vi "Handle Command.vi"(8 "error in (no error)":errorcluster, 9 "Data":variant, 10 "Command":string, 11 "Inst.TSL210 in":refnum<class "Inst.TSL210.lvclass">) -> (0 "error out":errorcluster, 1 "Processed Data":variant, 2 "Command":string, 3 "Inst.TSL210 out":refnum<class "Inst.TSL210.lvclass">)   [LabVIEW 2019, in "Inst.TSL210.lvclass"]
uses:
  Inst.TSL210.lvclass
  Inst.TSL210.lvclass/Inst.TSL210.ctl
  <userlib>/LevyLab/Instrument Framework/Instrument Types/VSource/Instrument.VSource.lvclass
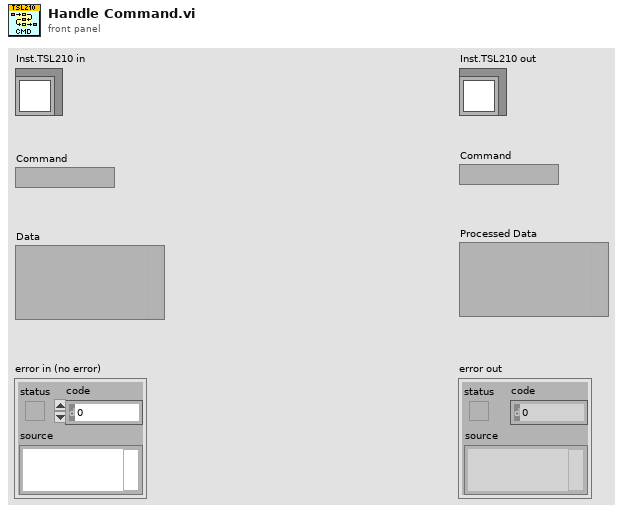
[diagram p1: front panel]
types:
  T1 = typedef "Inst.TSL210.lvclass/Inst.TSL210.getAll--Cluster.ctl" = cluster{"Wavelength (nm)":dbl, "Power (mW)":dbl, "Status: LD":bool, "Status: COH":bool, "Status: TempError":bool, "Status: CurrentLimit":bool, "Status: SystemBusy":bool, "Status: ATT":bool, "Status: ACC":bool, "Status: FT":bool}
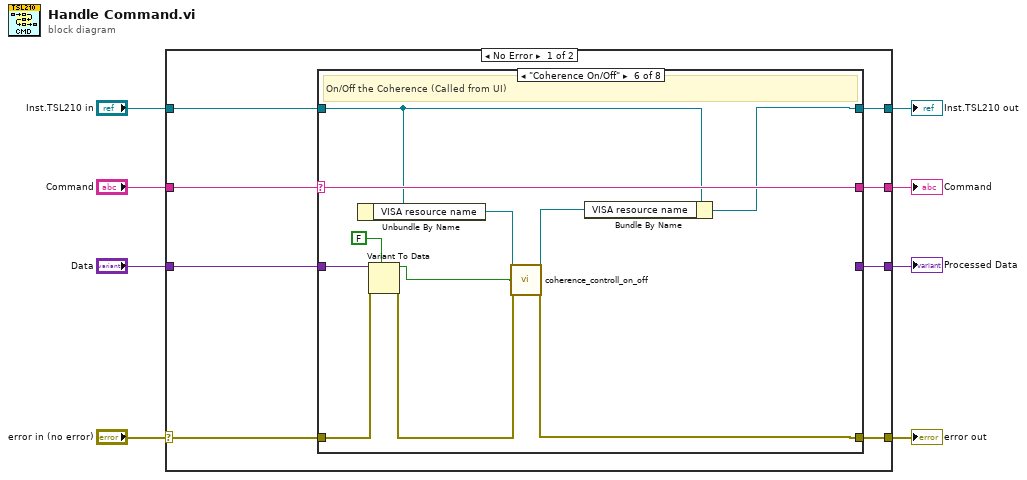
[diagram p0: block diagram]
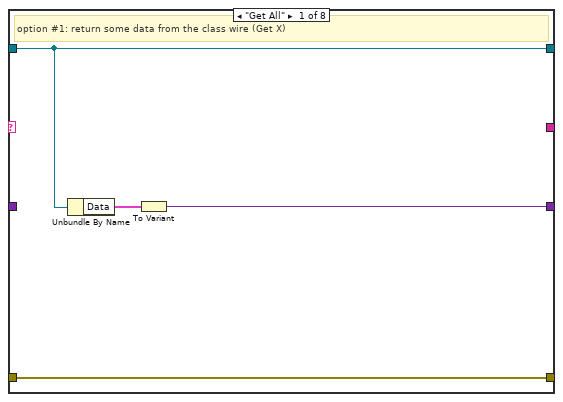
[diagram p2: hidden frame]
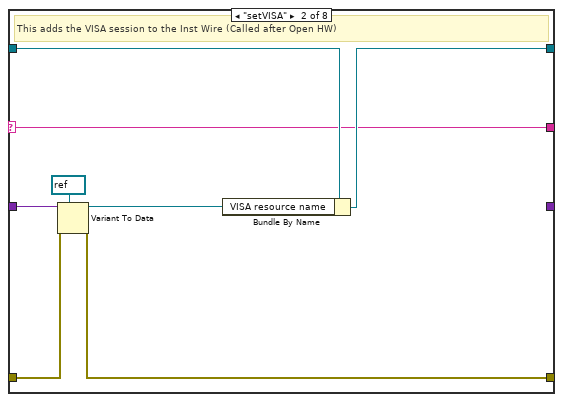
[diagram p3: hidden frame]
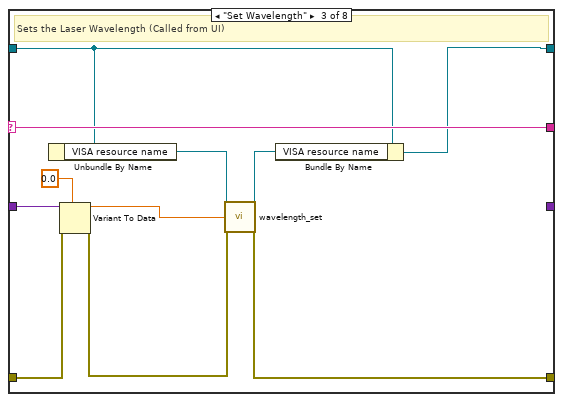
[diagram p4: hidden frame]
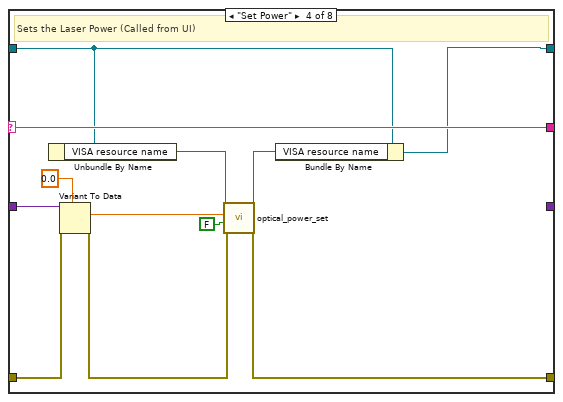
[diagram p5: hidden frame]
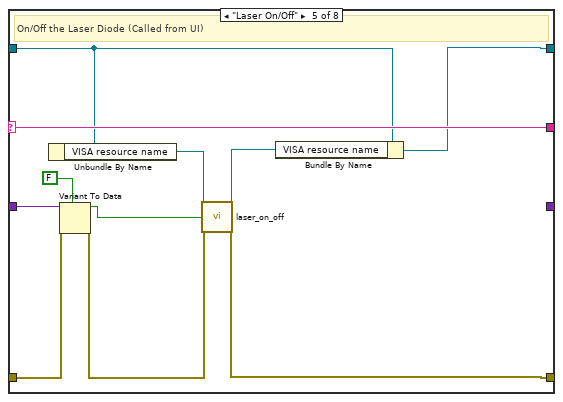
[diagram p6: hidden frame]
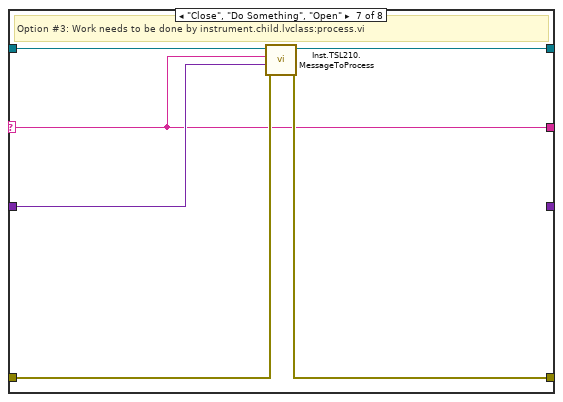
[diagram p7: hidden frame]
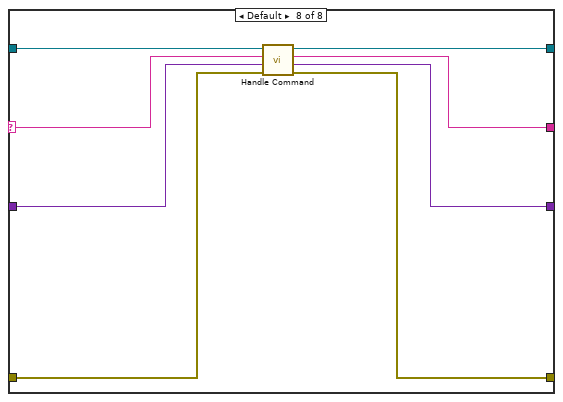
[diagram p8: hidden frame]
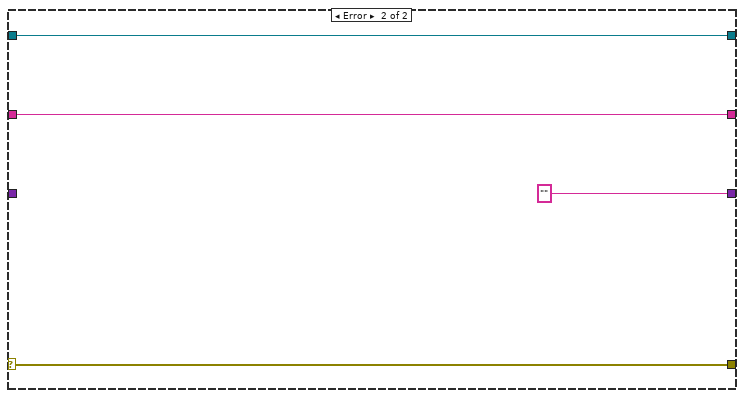
[diagram p9: hidden frame]
diagram:
  n1 = case shown="No Error" "error in (no error)" {
    selector: "error in (no error)" -> [w10 w91]
    tunnel: [w12 w91] -> w6
    tunnel: [w14 w90] -> w5
    tunnel: "Inst.TSL210 in" -> [w15 w90]
    tunnel: "Command" -> [w16 w88]
    tunnel: [w13 "" ("String")] -> w3
    tunnel: "Data" -> [w9 _]
    tunnel: [w11 w88] -> w1
    frame No Error {
      n2 = case shown="\"Coherence On/Off\"" w16 {
        selector: w16 -> [_ w26 w39 w51 w62 w73 w74 w81]
        tunnel: w15 -> [w19 w28 w31 w47 w59 w70 w79 w85]
        tunnel: [w19 w27 w30 w46 w58 w69 w78 w82] -> w14
        tunnel: [w17 _ _ _ _ _ _ w84] -> w13
        tunnel: w10 -> [w18 w24 w37 w49 w60 w71 w77 w86]
        tunnel: w9 -> [_ w25 w38 w50 w61 w72 w75 w87]
        tunnel: [w18 w23 w32 w45 w55 w66 w76 w83] -> w12
        tunnel: [_ w26 w39 w51 w62 w73 w74 w80] -> w11
        frame "Get All" {
          # "option #1: return some data from the class wire (Get X)"
          n3 = Unbundle By Name(w19) -> ("Data"=w20:T1)
          n4 = To Variant(anything=w20) -> (Variant=w17:variant)
        }
        frame "setVISA" {
          # "This adds the VISA session to the Inst Wire (Called after Open HW)"
          n5 = Variant To Data(error in=w24, type=refnum<visa-resource-name> refnum ("VISA resource name"), Variant=w25) -> (data=w21:refnum<visa-resource-name>, error out=w23:errorcluster)
          n6 = Bundle By Name(cluster=w28, "VISA resource name"=w21) -> (w27:refnum<class "Inst.TSL210.lvclass">)
        }
        frame "Set Wavelength" {
          # "Sets the Laser Wavelength (Called from UI)"
          n7 = Unbundle By Name(w31) -> ("VISA resource name"=w35:refnum<visa-resource-name>)
          n8 = Variant To Data(error in=w37, type=0.0, Variant=w38) -> (data=w34:dbl, error out=w33:errorcluster)
          n9 = call "wavelength_set.vi"("error in (no error)"=w33, "Wavelength in nm"=w34, "VISA session (for class)"=w35) -> ("error out"=w32:errorcluster, "dup VISA session"=w29:refnum<visa-resource-name>)  [unwired: 1 out]
          n10 = Bundle By Name(cluster=w31, "VISA resource name"=w29) -> (w30:refnum<class "Inst.TSL210.lvclass">)
        }
        frame "Set Power" {
          # "Sets the Laser Power (Called from UI)"
          n11 = Unbundle By Name(w47) -> ("VISA resource name"=w41:refnum<visa-resource-name>)
          n12 = Variant To Data(error in=w49, type=0.0, Variant=w50) -> (data=w42:dbl, error out=w44:errorcluster)
          n13 = call "optical_power_set.vi"("error in (no error)"=w44, "unit dBM: TRUE\n        mW: FALSE"=FALSE ("unit dBM: TRUE\n        mW: FALSE"), "optical output power in UNIT"=w42, "VISA session (for class)"=w41) -> ("error out"=w45:errorcluster, "dup VISA session"=w40:refnum<visa-resource-name>)  [unwired: 1 out]
          n14 = Bundle By Name(cluster=w47, "VISA resource name"=w40) -> (w46:refnum<class "Inst.TSL210.lvclass">)
        }
        frame "Laser On/Off" {
          # "On/Off the Laser Diode (Called from UI)"
          n15 = Unbundle By Name(w59) -> ("VISA resource name"=w53:refnum<visa-resource-name>)
          n16 = Variant To Data(error in=w60, type=FALSE ("unit dBM: TRUE\n        mW: FALSE"), Variant=w61) -> (data=w52:bool, error out=w56:errorcluster)
          n17 = call "laser_on_off.vi"("error in (no error)"=w56, "Laser ON / OFF"=w52, "VISA session (for class)"=w53) -> ("error out"=w55:errorcluster, "dup VISA session"=w54:refnum<visa-resource-name>)  [unwired: 1 out]
          n18 = Bundle By Name(cluster=w59, "VISA resource name"=w54) -> (w58:refnum<class "Inst.TSL210.lvclass">)
        }
        frame "Coherence On/Off" {
          # "On/Off the Coherence (Called from UI)"
          n19 = Unbundle By Name(w70) -> ("VISA resource name"=w64:refnum<visa-resource-name>)
          n20 = Variant To Data(error in=w71, type=FALSE ("unit dBM: TRUE\n        mW: FALSE"), Variant=w72) -> (data=w63:bool, error out=w67:errorcluster)
          n21 = call "coherence_controll_on_off.vi"("error in (no error)"=w67, "Coherence Controll\n ON / OFF"=w63, "VISA session (for class)"=w64) -> ("error out"=w66:errorcluster, "dup VISA session"=w65:refnum<visa-resource-name>)  [unwired: 1 out]
          n22 = Bundle By Name(cluster=w70, "VISA resource name"=w65) -> (w69:refnum<class "Inst.TSL210.lvclass">)
        }
        frame "Close", "Do Something", "Open" {
          # "Option #3: Work needs to be done by instrument.child.lvclass:process.vi"
          n23 = call "Inst.TSL210.MessageToProcess.vi"("error in (no error)"=w77, "Data"=w75, "Command"=w74, "Inst.TSL210 in"=w79) -> ("error out"=w76:errorcluster, "Inst.TSL210 out"=w78:refnum<class "Inst.TSL210.lvclass">)  [unwired: 6 in]
        }
        frame Default {
          n24 = call-parent "Handle Command.vi"("error in (no error)"=w86, "Data"=w87, "Command"=w81, "Instrument in"=w85) -> ("error out"=w83:errorcluster, "Processed Data"=w84:variant, "Command"=w80:string, "Instrument out"=w82:refnum<class "Inst.TSL210.lvclass">)  [unwired: 4 in]
        }
      }
    }
    frame Error {
    }
  }
  "error out" <- w6
  "Inst.TSL210 out" <- w5
  "Command" <- w1
  "Processed Data" <- w3
